vi "ExtractSectionsFromString.vi"(11 "String":string) -> (2 "Sections":cluster{"key":string, "value":string}[](array[cluster]), 3 "String dup":string)   [LabVIEW 2013, in "Serializer.PlainText.INI.lvclass"]
uses:
  Serializer.PlainText.INI.lvclass
  <vilib>/regexp/Match Regular Expression.xnode
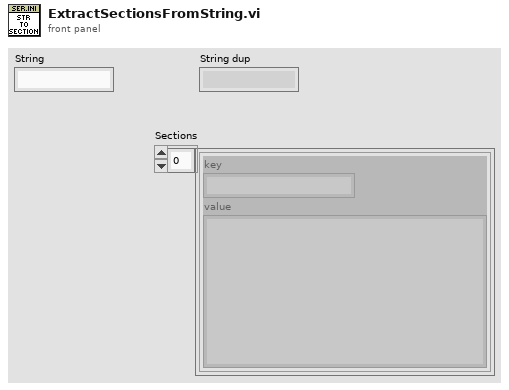
[diagram p1: front panel]
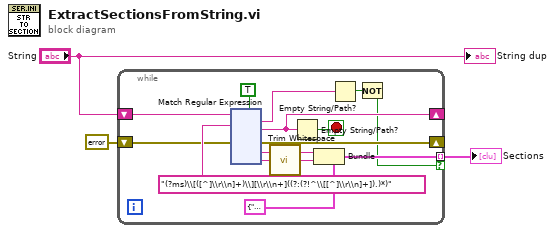
[diagram p0: block diagram]
diagram:
  n1 = while {
    shift-right: [w12] -> _
    shift-left: "String" -> [w18]
    tunnel: [w13] -> w3 mode=indexing if=w6
    shift-right: [w10] -> _
    shift-left: errorcluster {"status"=FALSE, "code"=0, "source"=""} ("error out") -> [w9]
    stop <- w11 stop-if-true
    n2 = xnode "Match Regular Expression"("input string"=w18, "regular expression"="(?ms)\\[([^]\\r\\n]+)\\][\\r\\n+]((?:(?!^\\[[^]\\r\\n]+]).)*)" ("input string"), "error in"=w9, "multiline? (F)"=TRUE) -> ("whole match"=w4:string, "after match"=w12:string, "error out"=w10:errorcluster, "submatch 1"=w16:string, "submatch 2"=w15:string)  [unwired: 2 in, 2 out]
    n3 = call <vilib>:"Trim Whitespace.vi"("string"=w15) -> ("trimmed string"=w14:string)  [unwired: 1 in]
    n4 = Empty String/Path?(string/path=w12) -> (empty?=w11:bool)
    n5 = Bundle(cluster=cluster{"key":string, "value":string} {"key"="", "value"=""}, "key"=w16, "value"=w14) -> (w13:cluster{"key":string, "value":string})
    n6 = Empty String/Path?(string/path=w4) -> (empty?=w7:bool)
    n7 = Not(x=w7) -> (.not. x?=w6:bool)
  }
  "Sections" <- w3
  "String dup" <- "String"
